vi "Extract Gemini Response.vi"(0 "headers":string, 5 "body":string, 11 "error in":errorcluster) -> (4 "value":string, 15 "error out":errorcluster)   [LabVIEW 2020, in "llm_gemini_chatmodels.lvclass"]
uses:
  llm_gemini_chatmodels.lvclass
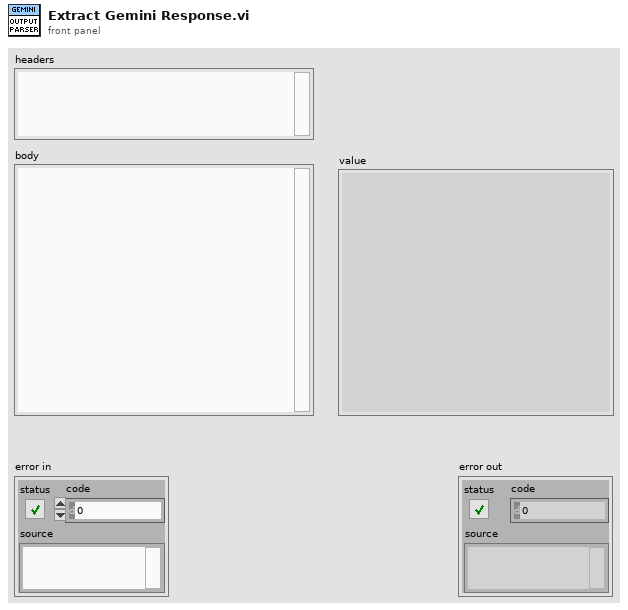
[diagram p1: front panel]
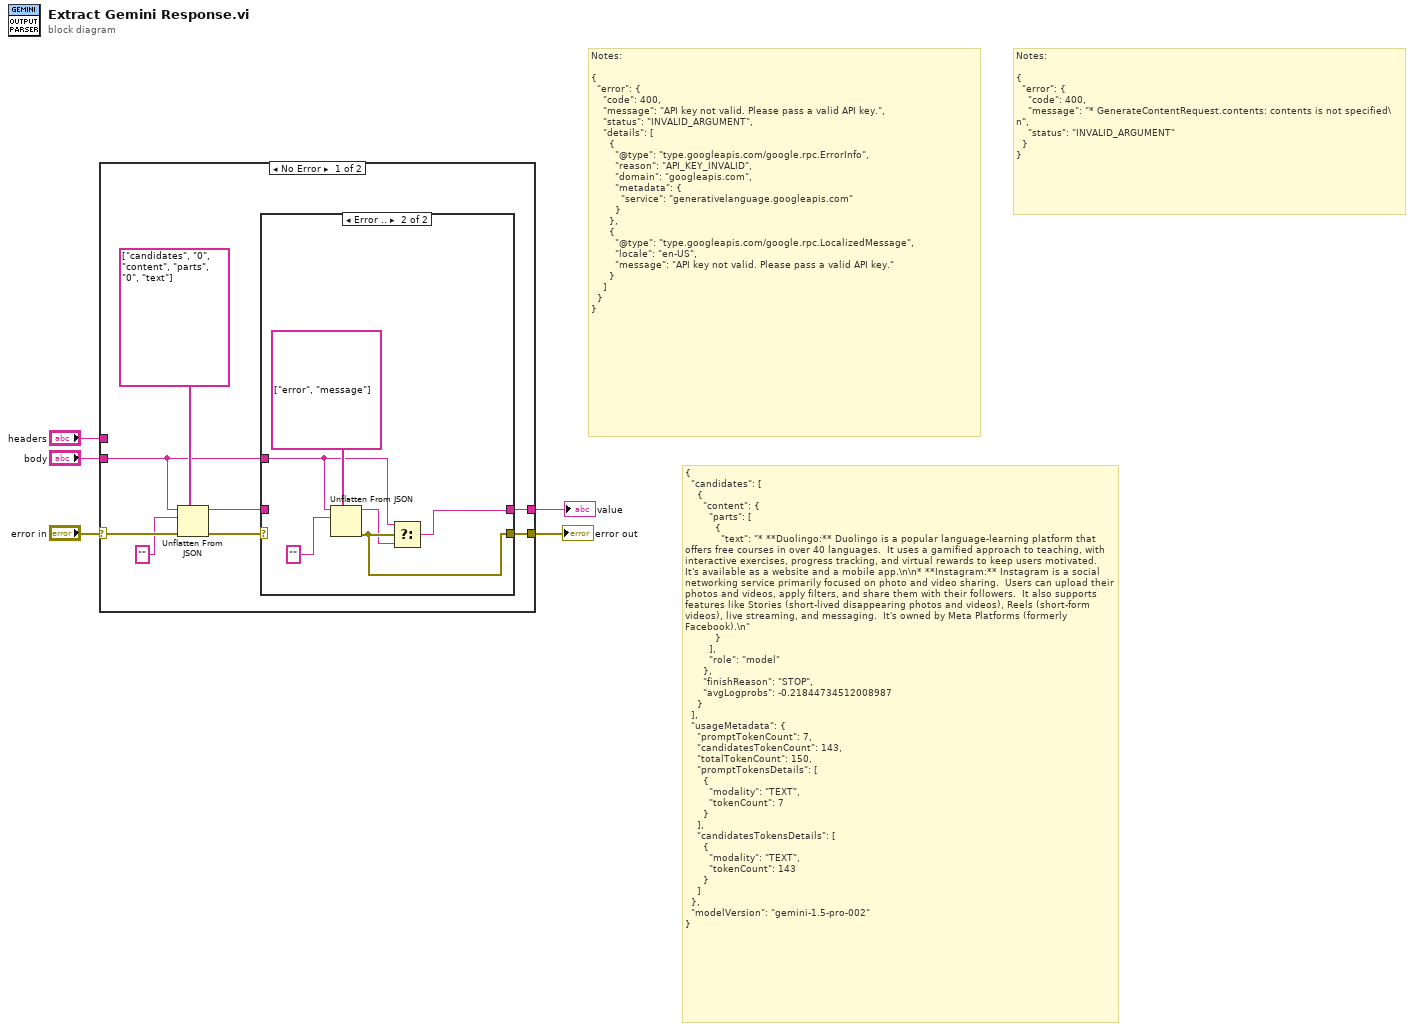
[diagram p0: block diagram]
diagram:
  # "Notes:\n\n{\n  \"error\": {\n    \"code\": 400,\n    \"message\": \"* GenerateContentRequest.contents: contents is not specified\\n\",\n    \"status\": \"INVALID_ARGUMENT\"\n  }\n}"
  # "{\n  \"candidates\": [\n    {\n      \"content\": {\n        \"parts\": [\n          {\n            \"text\": \"* **Duolingo:** Duolingo is a popular language-learning platform that offers free courses in over 40 languages.  It uses a gamified approach to teaching, with interactive exercises, progress tracking, and virtual rewards to keep users motivated.  It's available as a website and a mobile app.\\n\\n* **Instagram:** Instagram is a social networking service primarily focused on photo and video sharing.  Users can upload their photos and videos, apply filters, and share them with their followers.  It also supports features like Stories (short-lived disappearing photos and videos), Reels (short-form videos), live streaming, and messaging.  It's owned by Meta Platforms (formerly Facebook).\\n\"\n          }\n        ],\n        \"role\": \"model\"\n      },\n      \"finishReason\": \"STOP\",\n      \"avgLogprobs\": -0.21844734512008987\n    }\n  ],\n  \"usageMetadata\": {\n    \"promptTokenCount\": 7,\n    \"candidatesTokenCount\": 143,\n    \"totalTokenCount\": 150,\n    \"promptTokensDetails\": [\n      {\n        \"modality\": \"TEXT\",\n        \"tokenCount\": 7\n      }\n    ],\n    \"candidatesTokensDetails\": [\n      {\n        \"modality\": \"TEXT\",\n        \"tokenCount\": 143\n      }\n    ]\n  },\n  \"modelVersion\": \"gemini-1.5-pro-002\"\n}"
  # "Notes:\n\n{\n  \"error\": {\n    \"code\": 400,\n    \"message\": \"API key not valid. Please pass a valid API key.\",\n    \"status\": \"INVALID_ARGUMENT\",\n    \"details\": [\n      {\n        \"@type\": \"type.googleapis.com/google.rpc.ErrorInfo\",\n        \"reason\": \"API_KEY_INVALID\",\n        \"domain\": \"googleapis.com\",\n        \"metadata\": {\n          \"service\": \"generativelanguage.googleapis.com\"\n        }\n      },\n      {\n        \"@type\": \"type.googleapis.com/google.rpc.LocalizedMessage\",\n        \"locale\": \"en-US\",\n        \"message\": \"API key not valid. Please pass a valid API key.\"\n      }\n    ]\n  }\n}"
  n1 = case shown="No Error" "error in" {
    selector: "error in" -> [w13 w23]
    tunnel: [w9 w23] -> w4
    tunnel: "body" -> [w8 _]
    tunnel: "headers" -> [_ w22]
    tunnel: [w6 w22] -> w1
    frame No Error {
      n2 = Unflatten From JSON(path=string[] ["candidates", "0", "content", "parts", "0", "text"], JSON string=w8, type and defaults="", error in (no error)=w13) -> (value=w7:string, error out=w10:errorcluster)  [unwired: 3 in]
      n3 = case shown="Error .." w10 {
        selector: w10 -> [w15 _]
        tunnel: [w15 w18] -> w9
        tunnel: w8 -> [_ w16]
        tunnel: w7 -> [w14 _]
        tunnel: [w14 w19] -> w6
        frame No Error {
        }
        frame Error {
          n4 = Unflatten From JSON(path=string[] ["error", "message"], JSON string=w16, type and defaults="") -> (value=w17:string, error out=w18:errorcluster)  [unwired: 4 in]
          n5 = Select(t=w16, s=w18, f=w17) -> (s? t:f=w19:string)
        }
      }
    }
    frame Error {
    }
  }
  "error out" <- w4
  "value" <- w1
